vi "DAQmx Write (Analog 1D DBL NChan 1Samp).vi"(0 "task/channels in":refnum<k21>, 1 "auto start":bool=TRUE, 7 "data":dbl[](array[numeric]) format="%0.2f", 9 "timeout":dbl=10.0 format="%0.2f", 11 "error in":errorcluster) -> (4 "task out":refnum<k21>, 10 "number of samples written per channel":u32, 15 "error out":errorcluster)   [LabVIEW 2013]
doc: "Writes a single floating-point sample to each channel in a task that contains one or more analog output channels."
uses:
  nilvaiu.dll
panel:
  # "channel"
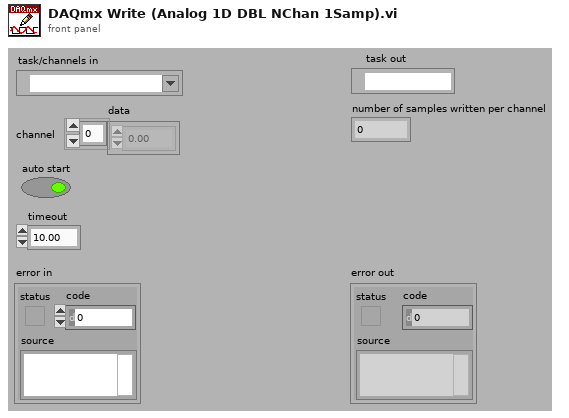
[diagram p1: front panel]
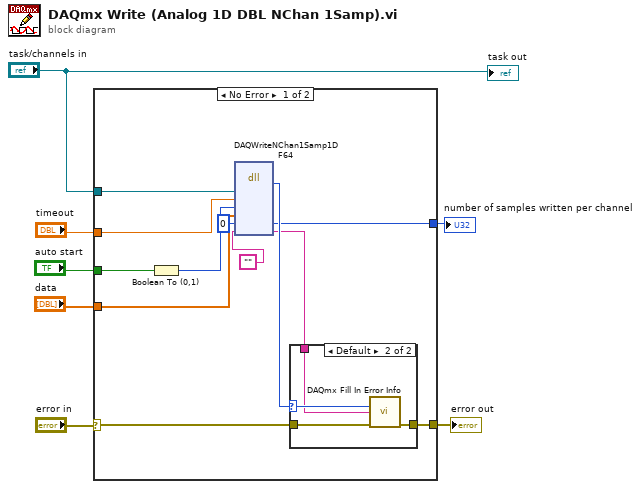
[diagram p0: block diagram]
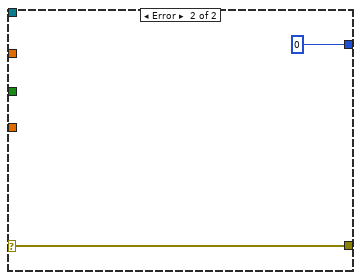
[diagram p3: hidden frame]
diagram:
  n1 = case shown="No Error" "error in" {
    selector: "error in" -> [w11 w25]
    tunnel: [w17 w25] -> w5
    tunnel: "task/channels in" -> [w19 _]
    tunnel: [w12 u32 0 ("numSamplesWriten")] -> w4
    tunnel: "timeout" -> [w10 _]
    tunnel: "auto start" -> [w9 _]
    tunnel: "data" -> [w8 _]
    frame No Error {
      n2 = Boolean To (0,1)(Boolean=w9) -> (0, 1=w16:i16)
      n3 = dll-call lib="nilvaiu.*" fn="DAQWriteNChan1Samp1DF64"("taskID"=w19, "timeout"=w10, "autoStart"=w16, "data"=w8, "numSamplesWriten"=u32 0, "extendedErrorInfo"="") -> (w18:i32, "numSamplesWriten"=w12:u32, "extendedErrorInfo"=w14:string)  [unwired: 5 in, 4 out]
      n4 = case shown="Default" w18 {
        selector: w18 -> [_ w22]
        tunnel: w11 -> [w20 w24]
        tunnel: [w20 w23] -> w17
        tunnel: w14 -> [_ w21]
        frame 0 {
        }
        frame Default {
          n5 = call "DAQmx Fill In Error Info.vi"("status code"=w22, "extended error info"=w21, "error in"=w24) -> ("error out"=w23:errorcluster)  [unwired: 1 in, 11 out]
        }
      }
    }
    frame Error {
    }
  }
  "error out" <- w5
  "number of samples written per channel" <- w4
  "task out" <- "task/channels in"
